vi "Convert To Volts.vi"(8 "error in (no error)":errorcluster, 10 "Raw Data":i32[](array[numeric]), 11 "DataReceiver in":refnum<class "DataReceiver.lvclass">) -> (0 "error out":errorcluster, 2 "Volts":dbl[](array[numeric]), 3 "DataReceiver out":refnum<class "DataReceiver.lvclass">)   [LabVIEW 2010, in "DataReceiver.lvclass"]
uses:
  DataReceiver.lvclass
  DataReceiver.lvclass/DataReceiver.ctl
  <vilib>/Analysis/polynomials.llb/1D Polynomial Evaluation (DBL).vi
  <vilib>/Analysis/NI_AALPro.lvlib
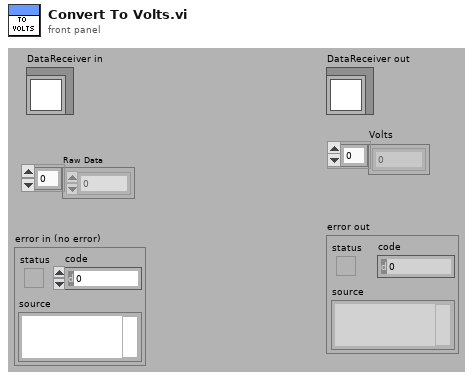
[diagram p1: front panel]
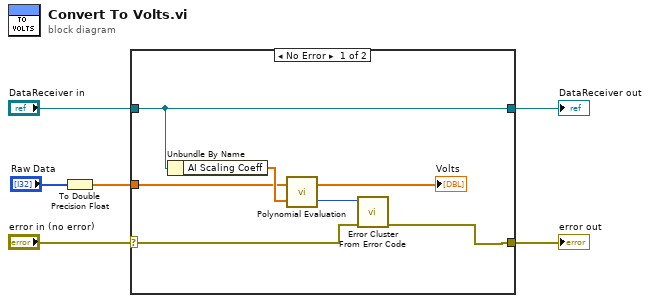
[diagram p0: block diagram]
diagram:
  n1 = To Double Precision Float(number="Raw Data") -> (double precision float=w1:dbl[])
  n2 = case shown="No Error" "error in (no error)" {
    selector: "error in (no error)" -> [w9 w15]
    tunnel: [w8 w15] -> w5
    tunnel: [w13 w14] -> w3
    tunnel: "DataReceiver in" -> [w13 w14]
    tunnel: w1 -> [w11 _]
    frame No Error {
      n3 = Unbundle By Name(w13) -> ("AI Scaling Coeff"=w12:dbl[])
      n4 = call-poly <vilib>:"Polynomial Evaluation.vi"("P(x)"=w12, "A"=w11) -> ("error"=w10:i32, "P(A)"=→"Volts":dbl[])
      n5 = call <vilib>:"Error Cluster From Error Code.vi"("error in (no error)"=w9, "error code (0)"=w10) -> ("error out"=w8:errorcluster)  [unwired: 7 in]
    }
    frame Error {
    }
  }
  "error out" <- w5
  "DataReceiver out" <- w3
